vi "Trim Both Whitespace.vi"(0 "string":string) -> (2 "trimmed string":string)   [LabVIEW 2014, in "JKI-State-Machine-Plus.lvlib"]
doc: "Removes all ASCII white space (spaces, tabs, carriage returns, and linefeeds) from the beginning, end, or both ends of <B>string</B>. The Trim Whitespace VI does not remove double byte characters."
uses:
  JKI-State-Machine-Plus.lvlib
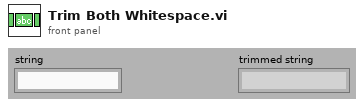
[diagram p1: front panel]
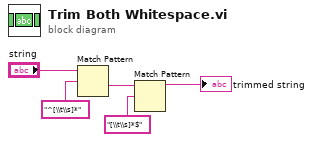
[diagram p0: block diagram]
diagram:
  n1 = Match Pattern(string="string", regular expression="^[\\t\\s]*") -> (after substring=w3:string)  [unwired: 1 in, 3 out]
  n2 = Match Pattern(string=w3, regular expression="[\\t\\s]*$") -> (before substring=→"trimmed string":string)  [unwired: 1 in, 3 out]
